vi "Read CommandStartTime.vi"(8 "error in (no error)":errorcluster, 11 "Command in":refnum<class "Command State Actor.lvclass">) -> (0 "error out":errorcluster, 2 "CommandStartTime":timestamp, 3 "Command out":refnum<class "Command State Actor.lvclass">)   [LabVIEW 2013, in "Command State Actor.lvlib" / "Command State Actor.lvclass"]
uses:
  Command State Actor.lvclass
  Command State Actor.lvclass/Command State Actor.ctl
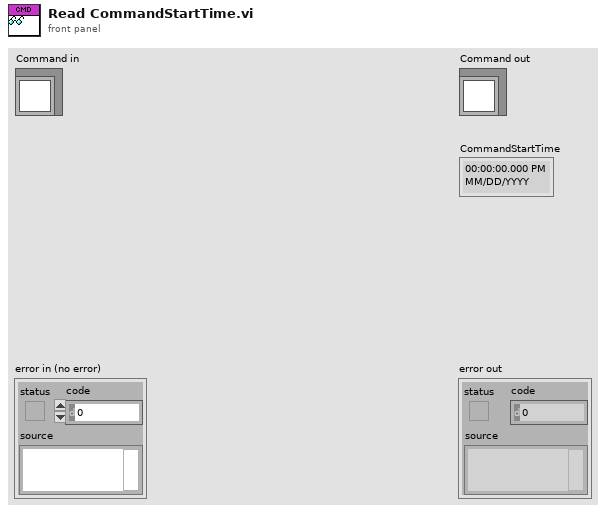
[diagram p1: front panel]
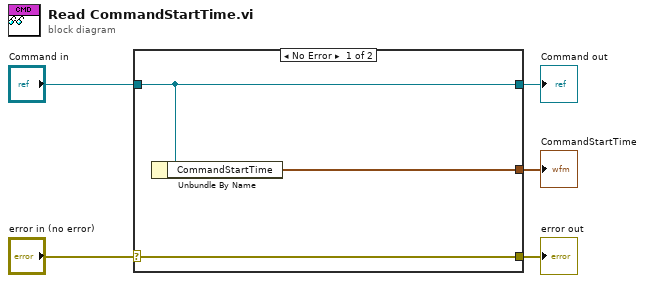
[diagram p0: block diagram]
diagram:
  n1 = case shown="No Error" "error in (no error)" {
    selector: "error in (no error)" -> [w8 w9]
    tunnel: [w8 w9] -> w4
    tunnel: [w7 w10] -> w2
    tunnel: "Command in" -> [w7 w10]
    tunnel: [w6 _] -> w1
    frame No Error {
      n2 = Unbundle By Name(w7) -> ("CommandStartTime"=w6:timestamp)
    }
    frame Error {
    }
  }
  "error out" <- w4
  "Command out" <- w2
  "CommandStartTime" <- w1
